vi "ReadyToKick.vi"(0 "object in":refnum<class "KickToSkill.lvclass">, 1 "first call?":bool, 3 "dest_orientation":dbl, 4 "target gap":dbl[](array[numeric]), 5 "error in (no error)":errorcluster) -> (14 "object out":refnum<class "KickToSkill.lvclass">, 16 "kick":bool, 19 "error out":errorcluster)   [LabVIEW 2023, in "KickToSkill.lvclass"]
uses:
  KickToSkill.lvclass
panel:
  out "Boolean":bool
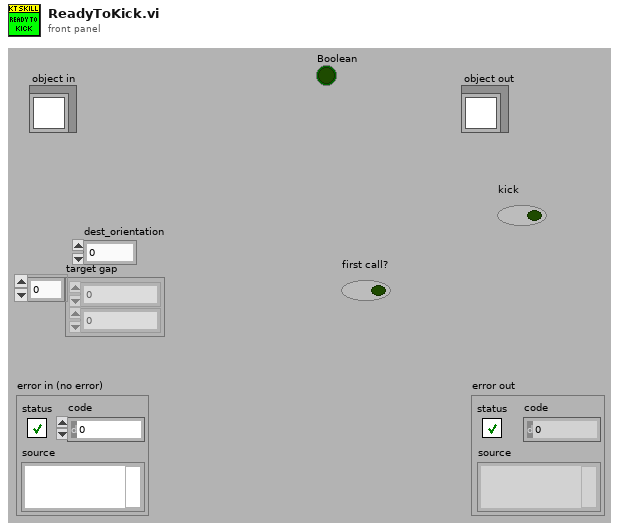
[diagram p1: front panel]
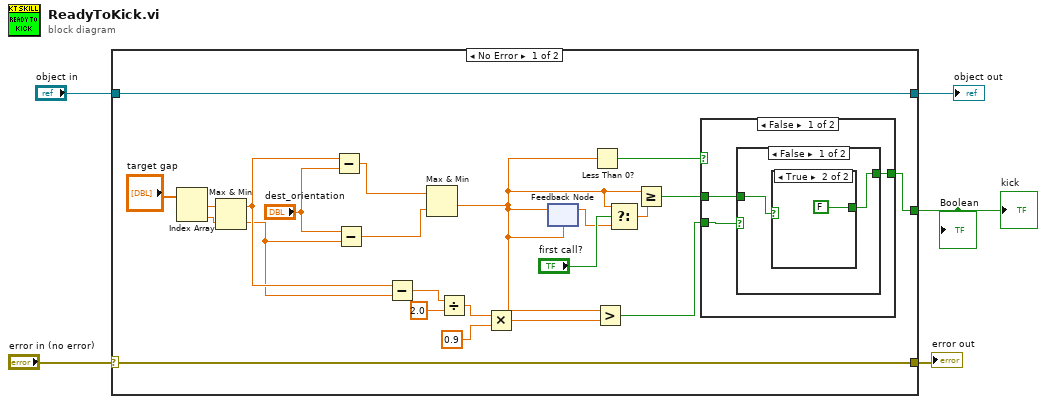
[diagram p0: block diagram]
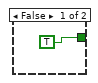
[diagram p2: hidden frame]
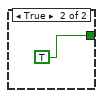
[diagram p3: hidden frame]
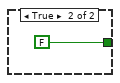
[diagram p4: hidden frame]
diagram:
  n1 = case shown="No Error" "error in (no error)" {
    selector: "error in (no error)" -> [w28 w39]
    tunnel: [w28 w39] -> w4
    tunnel: [w27 w38] -> w2
    tunnel: "object in" -> [w27 w38]
    tunnel: [w6 _] -> w1
    frame No Error {
      n2 = Index Array(array="target gap") -> (element #1=w11:dbl, element #2=w10:dbl)  [unwired: 2 in]
      n3 = Max & Min(x=w11, y=w10) -> (max(x,y)=w9:dbl, min(x,y)=w8:dbl)
      n4 = Subtract(x=w9, y="dest_orientation") -> (x-y=w13:dbl)
      n5 = Subtract(x="dest_orientation", y=w8) -> (x-y=w12:dbl)
      n6 = Subtract(x=w9, y=w8) -> (x-y=w24:dbl)
      n7 = Max & Min(x=w13, y=w12) -> (min(x,y)=w7:dbl)  [unwired: 1 out]
      n8 = Divide(x=w24, y=2.0) -> (x/y=w22:dbl)
      n9 = Multiply(x=w22, y=0.9) -> (x*y=w20:dbl)
      n10 = feedback-in #1(w7) -> ()
      n11 = feedback #1(w7) -> (w18:dbl)
      n12 = Less Than 0?(x=w7) -> (x < 0?=w16:bool)
      n13 = Greater?(x=w7, y=w20) -> (0:w15:bool)
      n14 = Select(t=w7, s="first call?", f=w18) -> (s? t:f=w17:dbl)
      n15 = Greater Or Equal?(x=w7, y=w17) -> (x >= y?=w14:bool)
      n16 = case shown="False" w16 {
        tunnel: [w30 FALSE] -> w6
        tunnel: w15 -> [w31 _]
        tunnel: w14 -> [w29 _]
        frame False {
          n17 = case shown="False" w31 {
            tunnel: [w32 TRUE] -> w30
            tunnel: w29 -> [w33 _]
            frame False {
              n18 = case shown="True" w33 {
                tunnel: [TRUE FALSE] -> w32
                frame False {
                }
                frame True {
                }
              }
            }
            frame True {
            }
          }
        }
        frame True {
        }
      }
    }
    frame Error {
    }
  }
  "error out" <- w4
  "object out" <- w2
  "kick" <- w1
  "Boolean" <- w1
